vi "ExCircGeoBufBin2x.vi"() -> ()   [LabVIEW 2010]
panel:
  in  "Rotate button":bool
  in  "Reverse button":bool
  in  "Flip button":bool
  in  "Intensifier":bool
  in  "Temperature":dbl=-10.0 format="%.2f"
  in  "Exposure":dbl min=0.0 step=0.001 format="%.3f"
  in  "stop":bool
  in  "Store":bool
  out "error out":errorcluster
  in  "error in (no error)":errorcluster
  # "ExCircGeoBufBin2x:\nThis example shows how to use the geometric online\noperations. This allows you to rotate, flip, or reverse\nthe image or any combnation of the 3. \nNote: This example uses circular buffers, not all \ncameras support circular buffers."
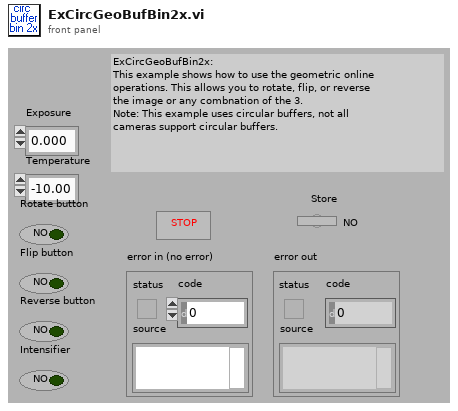
[diagram p1: front panel]
types:
  T1 = cluster{"acquire focus mode":u32, "Exposure":dbl, "Number of Images":u32, "Software accumulation":u32}
  T2 = cluster{"Camera Handle":u32, "Pulser Handle":u32, "File Handle":u32, "Display Handle":u32, "Image Handle":u32}
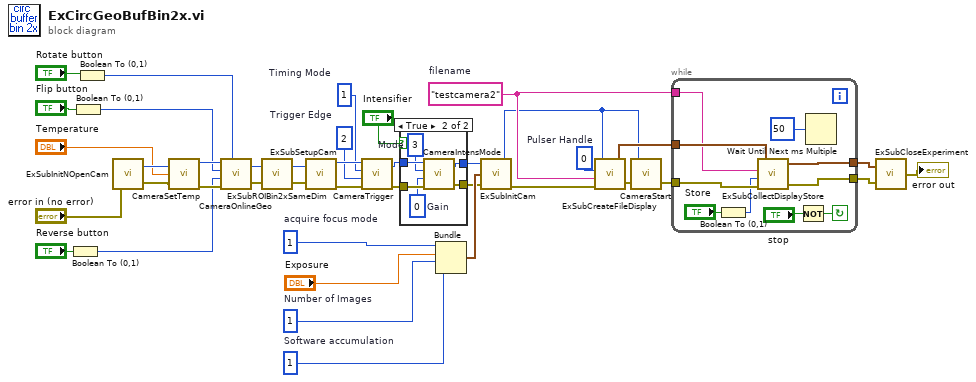
[diagram p0: block diagram]
diagram:
  w22 = u32 0  # Pulser Handle
  w23 = u32 1  # Timing Mode
  w24 = u32 2  # Trigger Edge
  w27 = u32 1  # acquire focus mode
  w26 = u32 1  # Number of Images
  w25 = u32 1  # Software accumulation
  w40 = "testcamera2"  # filename
  n1 = Boolean To (0,1)(Boolean="Reverse button") -> (0, 1=w2:i16)
  n2 = Boolean To (0,1)(Boolean="Flip button") -> (0, 1=w1:i16)
  n3 = Boolean To (0,1)(Boolean="Rotate button") -> (0, 1=w6:i16)
  n4 = call "ExSubInitNOpenCam.vi"("error in (no error)"="error in (no error)") -> ("Camera Handle"=w9:u32, "error out"=w8:errorcluster)
  n5 = call <userlib>:"CameraSetTemp.vi"("error in (no error)"=w8, "Temperature"="Temperature", "Camera Handle"=w9) -> ("error out"=w10:errorcluster, "Camera Handle"=w11:u32)
  n6 = call <userlib>:"CameraOnlineGeo.vi"("Camera Handle"=w11, "Flip Flag"=w1, "Reverse Flag"=w2, "error in"=w10, "Rotate Flag"=w6) -> ("Camera Handle"=w15:u32, "error out"=w14:errorcluster)
  n7 = call "ExSubROIBin2xSameDim.vi"("error in (no error)"=w14, "Camera Handle"=w15) -> ("error out"=w13:errorcluster, "Camera Handle"=w12:u32)
  n8 = call "ExSubSetupCam.vi"("error in (no error)"=w13, "Camera Handle"=w12) -> ("error out"=w30:errorcluster, "Camera Handle"=w31:u32)
  n9 = call <userlib>:"CameraTrigger.vi"("error in"=w30, "Trigger Edge"=w24, "Timing Mode"=w23, "Camera Handle"=w31) -> ("error out"=w18:errorcluster, "Camera Handle"=w20:u32)
  n10 = case shown="True" "Intensifier" {
    tunnel: w20 -> [w42 w48]
    tunnel: [w42 w47] -> w19
    tunnel: w18 -> [w41 w46]
    tunnel: [w41 w45] -> w17
    frame False {
    }
    frame True {
      w43 = u32 0  # Gain
      w44 = u32 3  # Mode
      n11 = call <userlib>:"CameraIntensMode.vi"("error in"=w46, "Intensifier Gain"=w43, "Mode"=w44, "Camera Handle"=w48) -> ("error out"=w45:errorcluster, "Camera Handle"=w47:u32)
    }
  }
  n12 = Bundle("acquire focus mode"=w27, "Exposure"="Exposure", "Number of Images"=w26, "Software accumulation"=w25) -> (w37:T1)  [unwired: 1 in]
  n13 = call "ExSubInitCam.vi"("error in (no error)"=w17, "Camera Information"=w37, "Camera Handle"=w19) -> ("error out"=w36:errorcluster, "Camera Handle"=w21:u32)
  n14 = call "ExSubCreateFileDisplay.vi"("error in (no error)"=w36, "File and Display Name"=w40, "Pulser Handle"=w22, "Camera Handle"=w21) -> ("error out"=w28:errorcluster, "Handles Out"=w35:T2)
  n15 = call <userlib>:"CameraStart.vi"("error in"=w28, "Camera Handle"=w21) -> ("error out"=w29:errorcluster)  [unwired: 1 out]
  n16 = while {
    tunnel: w35 -> [w57]
    tunnel: w29 -> [w56]
    tunnel: w40 -> [w49]
    tunnel: [w54] -> w33
    tunnel: [w55] -> w34
    stop <- w52 continue-if-true
    n17 = Boolean To (0,1)(Boolean="Store") -> (0, 1=w50:i16)
    n18 = call "ExSubCollectDisplayStore.vi"("error in (no error)"=w56, "Store flag"=w50, "Display Title"=w49, "Handle Cluster"=w57) -> ("error out"=w54:errorcluster, "Handle Cluster Out"=w55:T2)  [unwired: 1 out]
    n19 = Not(x="stop") -> (.not. x?=w52:bool)
    n20 = Wait Until Next ms Multiple(millisecond multiple=u32 50) -> ()  [unwired: 1 out]
  }
  n21 = call "ExSubCloseExperiment.vi"("error in (no error)"=w33, "Handles In"=w34) -> ("error out"=→"error out":errorcluster)
